vi "Create Main Files.vi"(11 "path":path) -> (1 "app.c":string, 2 "app.h":string, 3 "main.c":string)   [LabVIEW 2010]
uses:
  read_excel_values.llb/GetXL_CellValues_2D_String.vi
panel:
  out "error out":errorcluster
  # "Type: U8, I8, U16, I16, U32, I32, U64, I64, FLOAT"
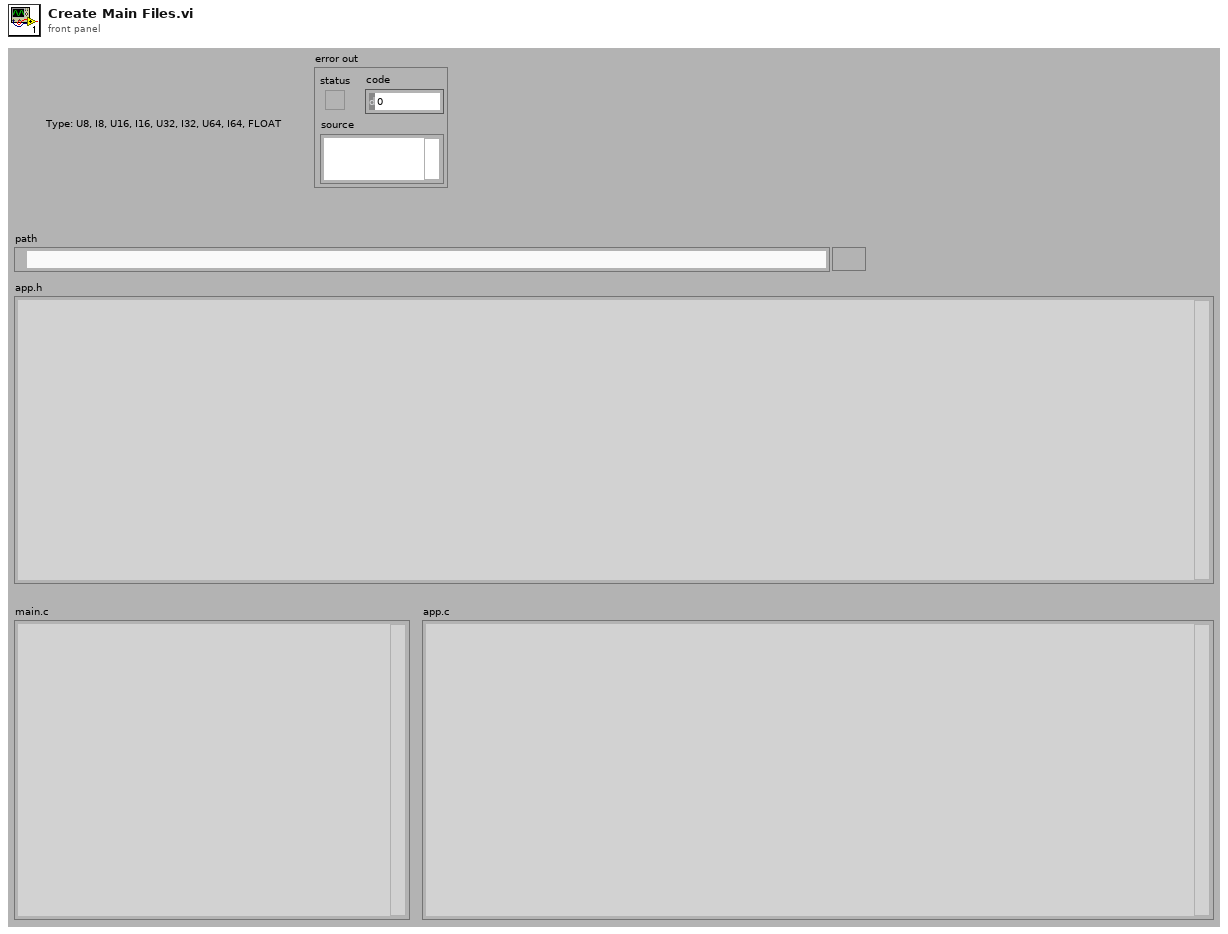
[diagram p1: front panel]
types:
  T1 = cluster{"Excel._Application":refnum<k7>, "Workbooks":refnum<k7>}
  T2 = cluster{"Excel._Application":refnum<k7>, "Workbooks":refnum<k7>, "Open":refnum<k7>}
  T3 = cluster{"Excel._Application":refnum<k7>, "Workbooks":refnum<k7>, "Open":refnum<k7>, "Worksheets":refnum<k7>, "Excel._Worksheet":refnum<k7>}
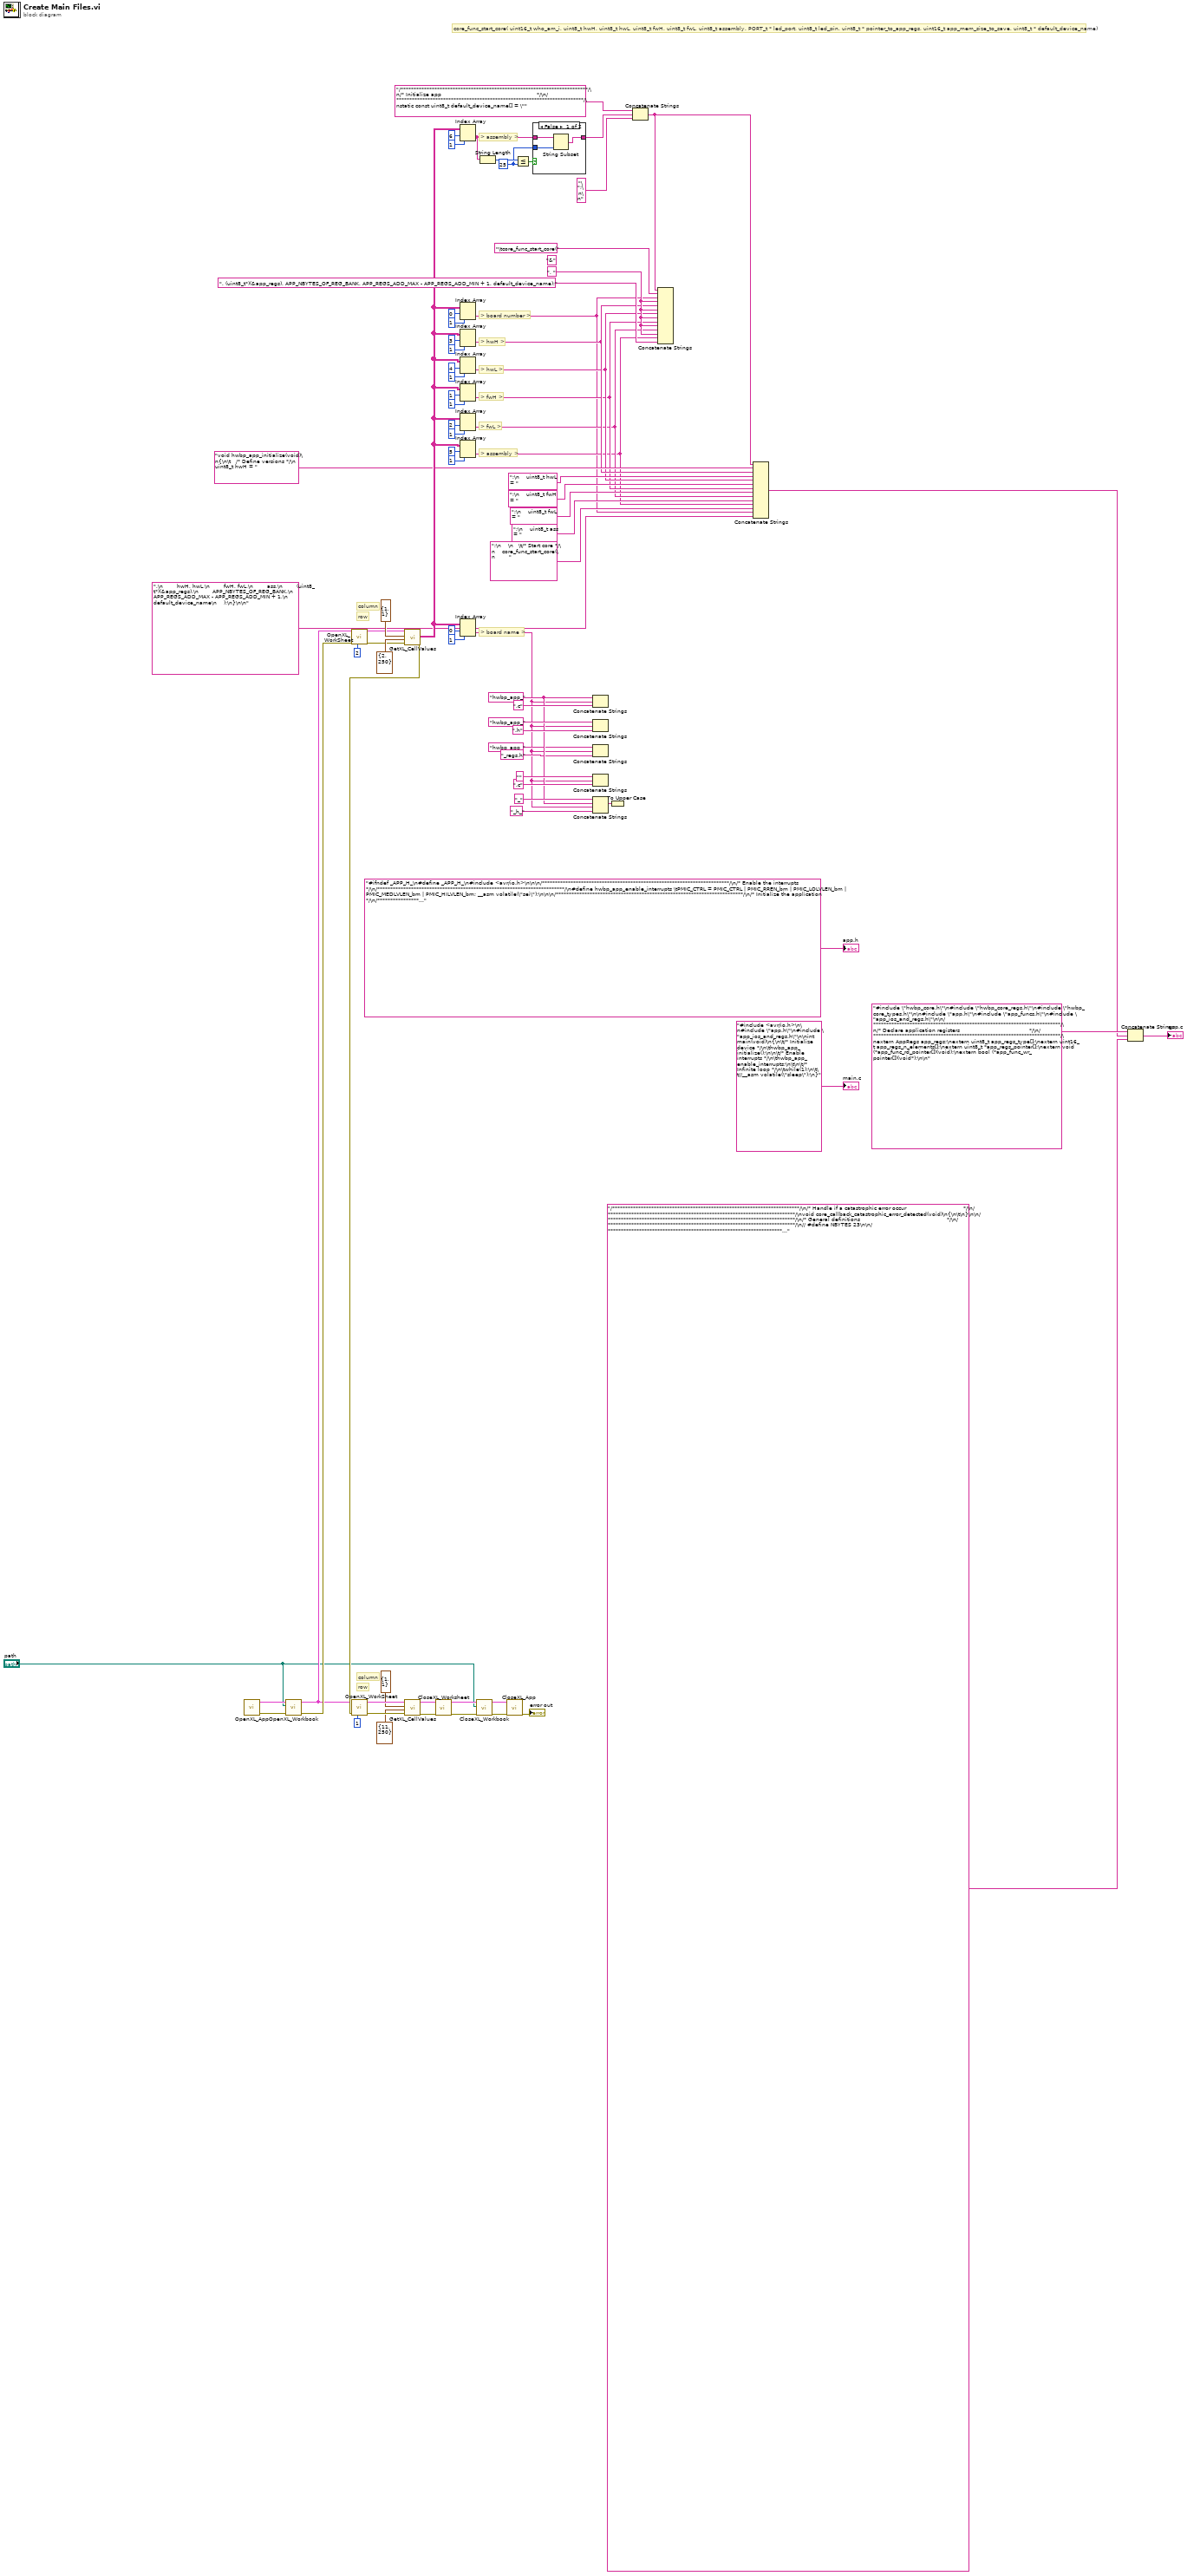
[diagram p0: block diagram]
diagram:
  w16 = 25 ("y")
  (unwired) "&" ("string")
  w30 = ", " ("string")
  w49 = "hwbp_app_" ("string")
  # "> assembly >"
  # "core_func_start_core( uint16_t who_am_i, uint8_t hwH, uint8_t hwL, uint8_t fwH, uint8_t fwL, uint8_t assembly, PORT_t * led_port, uint8_t led_pin, uint8_t * pointer_to_app_regs, uint16_t app_mem_size_to_save, uint8_t * default_device_name)"
  # "> assembly >"
  # "> fwL >"
  # "> fwH >"
  # "> hwL >"
  # "> hwH >"
  # "> board number >"
  # "> board name >"
  # "row"
  # "column"
  # "row"
  # "column"
  n1 = call "OpenXL_App.vi"() -> ("error out"=w74:errorcluster, "Refnum Cluster"=w75:T1)  [unwired: 10 in]
  n2 = call "OpenXL_Workbook.vi"("error in"=w74, "path"="path", "Refnum Cluster In"=w75) -> ("error out"=w60:errorcluster, "Refnum Cluster Out"=w58:T2)  [unwired: 7 in]
  n3 = call "OpenXL_WorkSheet.vi"("Sheet"=2, "error in (no error)"=w60, "Refnum Cluster In"=w58) -> ("error out"=w62:errorcluster, "Refnum Cluster Out"=w61:T3)  [unwired: 7 in]
  n4 = call-poly "GetXL_CellValues.vi"("error in"=w62, "End"=cluster{"Column":i32, "Row":i32} {"Column"=2, "Row"=250}, "Start"=cluster{"Column":i32, "Row":i32} {"Column"=1, "Row"=1}, "Refnum Cluster In"=w61) -> ("error out"=w59:errorcluster, "data"=w23:string[][])  [unwired: 5 in, 1 out]
  n5 = call "OpenXL_WorkSheet.vi"("Sheet"=1, "error in (no error)"=w59, "Refnum Cluster In"=w58) -> ("error out"=w81:errorcluster, "Refnum Cluster Out"=w82:T3)  [unwired: 7 in]
  n6 = call-poly "GetXL_CellValues.vi"("error in"=w81, "End"=cluster{"Column":i32, "Row":i32} {"Column"=11, "Row"=250}, "Start"=cluster{"Column":i32, "Row":i32} {"Column"=1, "Row"=1}, "Refnum Cluster In"=w82) -> ("error out"=w72:errorcluster, "Refnum Cluster Out"=w73:T3)  [unwired: 5 in, 1 out]
  n7 = call "CloseXL_Worksheet.vi"("error in (no error)"=w72, "Refnum Cluster In"=w73) -> ("error out"=w70:errorcluster, "Refnum Cluster Out"=w71:T2)  [unwired: 8 in]
  n8 = Index Array(array=w23, index (row)=6, index (col)=1 ("disabled index (col)")) -> (element=w18:string)
  n9 = Index Array(array=w23, index (row)=0, index (col)=1 ("disabled index (col)")) -> (element=w4:string)
  n10 = Index Array(array=w23, index (row)=3, index (col)=1 ("disabled index (col)")) -> (element=w14:string)
  n11 = Index Array(array=w23, index (row)=4, index (col)=1 ("disabled index (col)")) -> (element=w12:string)
  n12 = Index Array(array=w23, index (row)=1, index (col)=1 ("disabled index (col)")) -> (element=w10:string)
  n13 = Index Array(array=w23, index (row)=2, index (col)=1 ("disabled index (col)")) -> (element=w8:string)
  n14 = Index Array(array=w23, index (row)=5, index (col)=1 ("disabled index (col)")) -> (element=w6:string)
  n15 = Index Array(array=w23, index (row)=0, index (col)=1 ("disabled index (col)")) -> (element=w46:string)
  n16 = call "CloseXL_Workbook.vi"("error in (no error)"=w70, "path"="path", "Refnum Cluster In"=w71) -> ("error out"=w79:errorcluster, "Refnum Cluster Out"=w80:T1)  [unwired: 7 in]
  n17 = String Length(string=w18) -> (length=w20:i32)
  n18 = call "CloseXL_App.vi"("error in (no error)"=w79, "Refnum Cluster In"=w80) -> ("error out"=→"error out":errorcluster)  [unwired: 9 in]
  n19 = Less Or Equal?(x=w20, y=w16) -> (x <= y?=w19:bool)
  n20 = case shown="False" w19 {
    tunnel: w18 -> [w85 w86]
    tunnel: [w83 w86] -> w17
    tunnel: w16 -> [w84 _]
    frame False {
      n21 = String Subset(string=w85, length (rest)=w84) -> (substring=w83:string)  [unwired: 1 in]
    }
    frame True {
    }
  }
  n22 = Concatenate Strings(w49, w46, ".c" ("string")) -> ()  [unwired: 1 out]
  n23 = Concatenate Strings("hwbp_app_" ("string"), w46, ".h" ("string")) -> ()  [unwired: 1 out]
  n24 = Concatenate Strings("hwbp_app_" ("string"), w46, "_regs.h" ("string")) -> ()  [unwired: 1 out]
  n25 = Concatenate Strings("" ("string"), w46, ".c" ("string")) -> ()  [unwired: 1 out]
  n26 = Concatenate Strings("_" ("string"), w49, w46, "_h_" ("string")) -> (w51:string)
  n27 = To Upper Case(1:w51) -> ()  [unwired: 1 out]
  n28 = Concatenate Strings("/************************************************************************/\n/* Initialize app                                                       */\n/************************************************************************/\nstatic const uint8_t default_device_name[] = \"" ("string"), w17, "\";\n\n" ("string")) -> (w2:string)
  n29 = Concatenate Strings(w2, "\tcore_func_start_core(" ("string"), w4, w30, w14, w30, w12, w30, w10, w30, w8, w30, w6, ", (uint8_t*)(&app_regs), APP_NBYTES_OF_REG_BANK, APP_REGS_ADD_MAX - APP_REGS_ADD_MIN + 1, default_device_name);" ("string")) -> ()  [unwired: 1 out]
  n30 = Concatenate Strings(w2, "void hwbp_app_initialize(void)\n{\n\t   /* Define versions */\n    uint8_t hwH = " ("string"), w14, ";\n    uint8_t hwL = " ("string"), w12, ";\n    uint8_t fwH = " ("string"), w10, ";\n    uint8_t fwL = " ("string"), w8, ";\n    uint8_t ass = " ("string"), w6, ";\n    \n   \t/* Start core */\n    core_func_start_core(\n        " ("string"), w4, ",\n        hwH, hwL,\n        fwH, fwL,\n        ass,\n        (uint8_t*)(&app_regs),\n        APP_NBYTES_OF_REG_BANK,\n        APP_REGS_ADD_MAX - APP_REGS_ADD_MIN + 1,\n        default_device_name\n    );\n}\n\n" ("string")) -> (w1:string)
  n31 = Concatenate Strings("#include \"hwbp_core.h\"\n#include \"hwbp_core_regs.h\"\n#include \"hwbp_core_types.h\"\n\n#include \"app.h\"\n#include \"app_funcs.h\"\n#include \"app_ios_and_regs.h\"\n\n/************************************************************************/\n/* Declare application registers                                        */\n/************************************************************************/\nextern AppRegs app_regs;\nextern uint8_t app_regs_type[];\nextern uint16_t app_regs_n_elements[];\nextern uint8_t *app_regs_pointer[];\nextern void (*app_func_rd_pointer[])(void);\nextern bool (*app_func_wr_pointer[])(void*);\n\n" ("string"), w1, "/************************************************************************/\n/* Handle if a catastrophic error occur                                 */\n/************************************************************************/\nvoid core_callback_catastrophic_error_detected(void)\n{\n\t\n}\n\n/************************************************************************/\n/* General definitions                                                  */\n/************************************************************************/\n// #define NBYTES 23\n\n/************************************************************************/\n/* General used functions                                               */\n/************************************************************************/\n/* Load external functions if needed */\n//#include \"hwbp_app_pwm_gen_funcs.c\"\n\n/*\nvoid update_enabled_pwmx(void)\n{\n\tif (!core_bool_is_visual_enabled())\n\treturn;\n\t\n\tif (!(app_regs.REG_CH_CONFEN & B_USEEN0) || ((app_regs.REG_CH_CONFEN & B_USEEN0) && (app_regs.REG_CH_ENABLE & B_EN0)))\n\t\tset_ENABLED_PWM0;\n\telse\n\t\tclr_ENABLED_PWM0;\n}\n\nISR(PORTB_INT0_vect, ISR_NAKED)\n{\n\treti();\n}\n*/\n\n/************************************************************************/\n/* Initialization Callbacks                                             */\n/************************************************************************/\nvoid core_callback_1st_config_hw_after_boot(void)\n{\n\t/* Initialize IOs */\n\t/* Don't delete this function!!! */\n\tinit_ios();\n\t\n\t/* SYNC OUTx */\n\t//io_pin2out(&PORTC, 1, OUT_IO_DIGITAL, IN_EN_IO_DIS);\n\n\t/* TRIG_IN0 */\n\t//io_pin2in(&PORTF, 5, PULL_IO_TRISTATE, SENSE_IO_EDGES_BOTH);\n\t//io_set_int(&PORTF, INT_LEVEL_LOW, 0, (1<<5), true);\n}\n\nvoid core_callback_reset_registers(void)\n{\n\t/* Initialize registers */\n\t/*\n\tapp_regs.REG_CH0_FREQ = 10.0;\n\tapp_regs.REG_CH0_DUTYCYCLE = 50;\n\t\n\tif ((app_regs.REG_MODE0 & B_M0) == GM_USB_MODE)\n\t{\n\t\tapp_regs.REG_OUT0 = 0;\n\t}\n\n\tif ((app_regs.REG_MODE1AND2 & B_M1AND2) == GM_USB_MODE)\n\t{\n\t\tapp_regs.REG_OUT1 = 0;\n\t\tapp_regs.REG_OUT2 = 0;\n\t}\n\t*/\n}\n\nvoid core_callback_registers_were_reinitialized(void)\n{\n\t/* Check if the user indication is valid */\n\t//update_enabled_pwmx();\n\t\n\t/* Update state register */\n\t//app_regs.REG_TRIG_STATE = (read_TRIG_IN0) ? B_LTRG0 : 0;\n\t//app_regs.REG_TRIG_STATE |= (read_TRIG_IN1) ? B_LTRG1 : 0;\n\n\t/* Reset start bits */\n\t//app_regs.REG_TRG0_START = 0;\n\t//app_regs.REG_TRG1_START = 0;\n\n\t/*\n\tif ((app_regs.REG_MODE0 & B_M0) == GM_BNC_MODE)\n\t{\n\t\tapp_regs.REG_OUT0 = app_regs.REG_CTRL0;\n\t\tset_OUT0(app_regs.REG_OUT0);\n\t}\n\telse\n\t{\n\t\tset_OUT0(app_regs.REG_OUT0);\n\t}\n\t*/\n}\n\n/************************************************************************/\n/* Callbacks: Visualization                                             */\n/************************************************************************/\nvoid core_callback_visualen_to_on(void)\n{\n\t/* Update channels enable indicators */\n\t//update_enabled_pwmx();\n}\n\nvoid core_callback_visualen_to_off(void)\n{\n\t/* Clear all the enabled indicators */\n}\n\n/************************************************************************/\n/* Callbacks: Change on the operation mode                              */\n/************************************************************************/\nvoid core_callback_device_to_standby(void) {}\nvoid core_callback_device_to_active(void) {}\nvoid core_callback_device_to_enchanced_active(void) {}\nvoid core_callback_device_to_speed(void) {}\n\n/************************************************************************/\n/* Callbacks: 1 ms timer                                                */\n/************************************************************************/\nvoid core_callback_t_before_exec(void) {}\nvoid core_callback_t_after_exec(void) {}\nvoid core_callback_t_new_second(void) {}\nvoid core_callback_t_500us(void) {}\nvoid core_callback_t_1ms(void) {}\n\n/************************************************************************/\n/* Callbacks: uart control                                              */\n/************************************************************************/\nvoid core_callback_uart_rx_before_exec(void) {}\nvoid core_callback_uart_rx_after_exec(void) {}\nvoid core_callback_uart_tx_before_exec(void) {}\nvoid core_callback_uart_tx_after_exec(void) {}\nvoid core_callback_uart_cts_before_exec(void) {}\nvoid core_callback_uart_cts_after_exec(void) {}\n\n/************************************************************************/\n/* Callbacks: Read app register                                         */\n/************************************************************************/\nbool core_read_app_register(uint8_t add, uint8_t type)\n{\n\t/* Check if it will not access forbidden memory */\n\tif (add < APP_REGS_ADD_MIN || add > APP_REGS_ADD_MAX)\n\t\treturn false;\n\t\n\t/* Check if type matches */\n\tif (app_regs_type[add-APP_REGS_ADD_MIN] != type)\n\t\treturn false;\n\t\n\t/* Receive data */\n\t(*app_func_rd_pointer[add-APP_REGS_ADD_MIN])();\t\n\n\t/* Return success */\n\treturn true;\n}\n\n/************************************************************************/\n/* Callbacks: Write app register                                        */\n/************************************************************************/\nbool core_write_app_register(uint8_t add, uint8_t type, uint8_t * content, uint16_t n_elements)\n{\n\t/* Check if it will not access forbidden memory */\n\tif (add < APP_REGS_ADD_MIN || add > APP_REGS_ADD_MAX)\n\t\treturn false;\n\t\n\t/* Check if type matches */\n\tif (app_regs_type[add-APP_REGS_ADD_MIN] != type)\n\t\treturn false;\n\n\t/* Check if the number of elements matches */\n\tif (app_regs_n_elements[add-APP_REGS_ADD_MIN] != n_elements)\n\t\treturn false;\n\n\t/* Process data and return false if write is not allowed or contains errors */\n\treturn (*app_func_wr_pointer[add-APP_REGS_ADD_MIN])(content);\n}" ("string")) -> (→"app.c":string)
  "app.h" <- "#ifndef _APP_H_\n#define _APP_H_\n#include <avr/io.h>\n\n\n/************************************************************************/\n/* Enable the interrupts                                                */\n/************************************************************************/\n#define hwbp_app_enable_interrupts \tPMIC_CTRL = PMIC_CTRL | PMIC_RREN_bm | PMIC_LOLVLEN_bm | PMIC_MEDLVLEN_bm | PMIC_HILVLEN_bm; __asm volatile(\"sei\");\n\n\n/************************************************************************/\n/* Initialize the application                                           */\n/************************************************************************/\nvoid hwbp_app_initialize(void);\n\n\n#endif /* _APP_H_ */" ("string")
  "main.c" <- "#include <avr/io.h>\n\n#include \"app.h\"\n#include \"app_ios_and_regs.h\"\n\nint main(void)\n{\n\t/* Initialize device */\n\thwbp_app_initialize();\n\n\t/* Enable interrupts */\n\thwbp_app_enable_interrupts;\n\t\n\t/* Infinite loop */\n\twhile(1);\n\t\t//__asm volatile(\"sleep\");\n}" ("string")
